vi "Get Name.vi"(8 "error in (no error)":errorcluster, 11 "Task Base in":refnum<class "Task Base.lvclass">) -> (0 "error out":errorcluster, 2 "Name":string, 3 "Task Base out":refnum<class "Task Base.lvclass">)   [LabVIEW 2023, in "HAL GOOP4.lvlib" / "Task Base.lvclass"]
uses:
  Task Base.lvclass
  Task Base.lvclass/Task Base.ctl
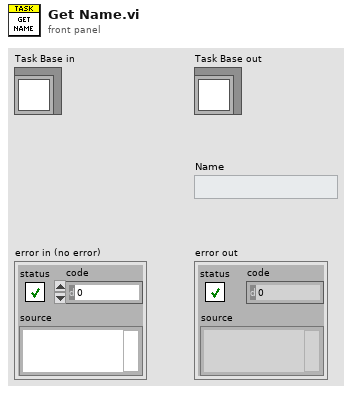
[diagram p1: front panel]
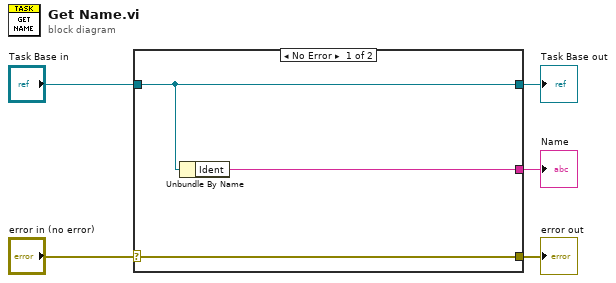
[diagram p0: block diagram]
diagram:
  n1 = case shown="No Error" "error in (no error)" {
    selector: "error in (no error)" -> [w8 w9]
    tunnel: [w8 w9] -> w4
    tunnel: [w7 w10] -> w2
    tunnel: "Task Base in" -> [w7 w10]
    tunnel: [w6 _] -> w1
    frame No Error {
      n2 = Unbundle By Name(w7) -> ("Ident"=w6:string)
    }
    frame Error {
    }
  }
  "error out" <- w4
  "Task Base out" <- w2
  "Name" <- w1
